vi "XNETInterfaceDiscover.vi"() -> (2 "CAN":cluster{"Interface":refnum<k21>[], "Slot":u32[]})   [LabVIEW 2018]
uses:
  FPGA Bitfiles/FPGA.ctl
  <resource>/objmgr/xnet.rc
panel:
  in  "FPGA VI (in)":T1
  out "iteration":i32
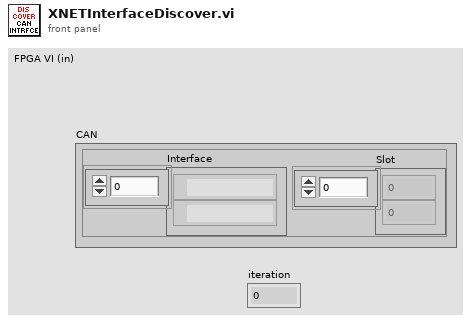
[diagram p1: front panel]
types:
  T1 = typedef "FPGA.ctl" = refnum<k20>
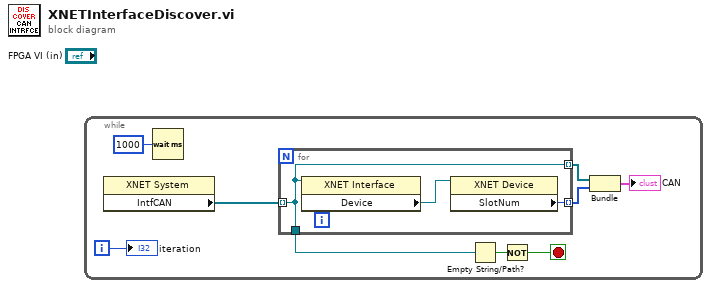
[diagram p0: block diagram]
diagram:
  n1 = while {
    i -> [w6]
    stop <- w4 stop-if-true
    n2 = property class="XNET System"() -> ("IntfCAN"=w9:refnum<k21>[])  [unwired: 2 in, 2 out]
    n3 = Wait (ms)(milliseconds to wait=u32 1000) -> ()  [unwired: 1 out]
    n4 = for {
      tunnel: w9 -> [w10] mode=indexing
      tunnel: [w10] -> w3 mode=indexing
      tunnel: [w11] -> w2 mode=indexing
      tunnel: [w10] -> w5
      n5 = property class="XNET Interface"(reference=w10) -> ("Device"=w12:refnum<k21>)  [unwired: 1 in, 2 out]
      n6 = property class="XNET Device"(reference=w12) -> ("SlotNum"=w11:u32)  [unwired: 1 in, 2 out]
    }
    n7 = Empty String/Path?(string/path=w5) -> (empty?=w7:bool)
    n8 = Not(x=w7) -> (.not. x?=w4:bool)
    n9 = Bundle(w3, w2) -> (→"CAN":cluster{refnum<k21>[], u32[]})  [unwired: 1 in]
    "iteration" <- w6
  }
